vi "GetText.vi"(8 "error in":errorcluster, 11 "Logic Sequencer editor node in":refnum<class "Logic Sequencer editor node.lvclass">) -> (0 "error out":errorcluster, 1 "additional text":string, 2 "text":string, 3 "Logic Sequencer editor node out":refnum<class "Logic Sequencer editor node.lvclass">, 4 "glyph":string)   [LabVIEW 2013, in "Logic Sequencer editor node.lvclass"]
uses:
  Logic Sequencer editor node.lvclass
  <vilib>/NI/Tag Bus Data Framework/Configuration Editor/Classes/Module editor node/Read display name.vi
  <vilib>/NI/Tag Bus Data Framework/Configuration Editor/PL Framework Configuration Tool.lvlib
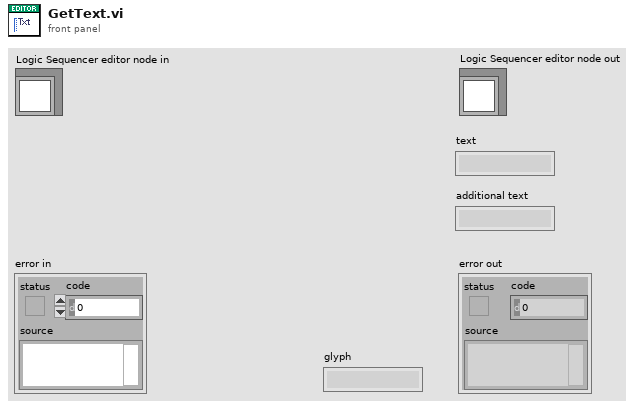
[diagram p1: front panel]
types:
  T1 = typedef "PL Framework Configuration Tool.lvlib/Glyphs Status.ctl" = enum16{"Normal", "Error", "Async"}
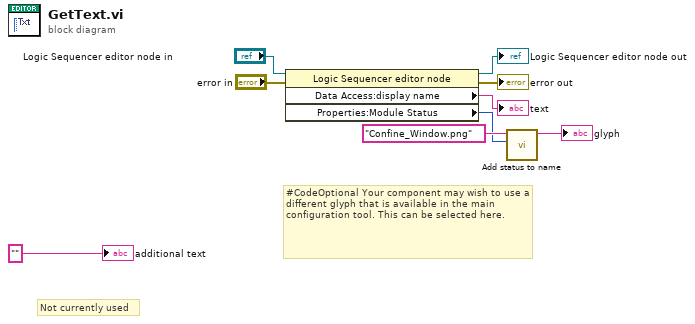
[diagram p0: block diagram]
diagram:
  # "Not currently used"
  # "#CodeOptional Your component may wish to use a different glyph that is available in the main configuration tool. This can be selected here."
  n1 = property class="Logic Sequencer editor node"(reference="Logic Sequencer editor node in", error in="error in") -> (reference out=→"Logic Sequencer editor node out":refnum<class "Logic Sequencer editor node.lvclass">, error out=→"error out":errorcluster, "Data Access:display name"=→"text":string, "Properties:Module Status"=w8:T1)
  n2 = call <vilib>:"Add status to name.vi"("Status"=w8, "Name"="Confine_Window.png" ("glyph")) -> ("Name with status"=→"glyph":string)  [unwired: 9 in]
  "additional text" <- "" ("additional text")
